vi "Query 1000.vi"(2 "error in (no error)":errorcluster, 3 "Parameters Query":T1) -> (0 "error out":errorcluster, 1 "Array":bool[](array[boolean]))   [LabVIEW 2015]
uses:
  C1G2_CommandControl.ctl
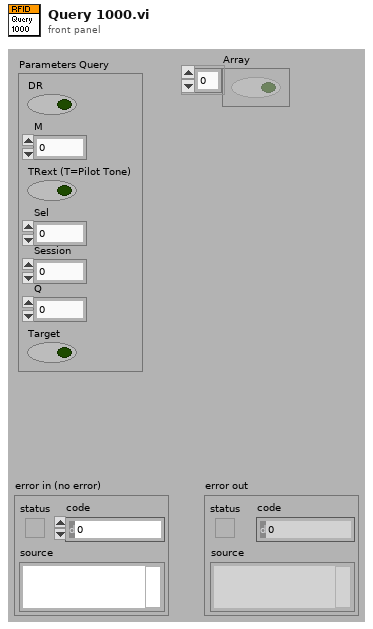
[diagram p1: front panel]
types:
  T1 = cluster{"DR":bool, "M":u16, "TRext (T=Pilot Tone)":bool, "Sel":u16, "Session":u16, "Q":u8, "Target":bool}
  T2 = typedef "C1G2_CommandControl.ctl" = u16
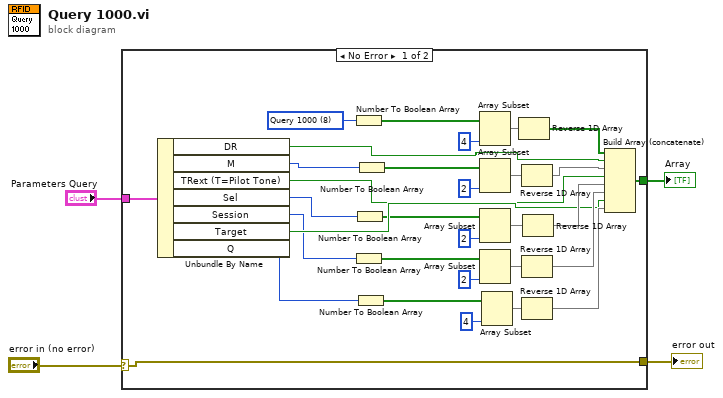
[diagram p0: block diagram]
diagram:
  n1 = case shown="No Error" "error in (no error)" {
    selector: "error in (no error)" -> [w5 w36]
    tunnel: [w35 _] -> w4
    tunnel: "Parameters Query" -> [w11 _]
    tunnel: [w5 w36] -> w1
    frame No Error {
      w6 = T2 8 items=["Select 1010"=10, "Query 1000"=8] ("Command")
      n2 = Unbundle By Name(w11) -> ("DR"=w14:bool, "M"=w7:u16, "TRext (T=Pilot Tone)"=w17:bool, "Sel"=w8:u16, "Session"=w9:u16, "Target"=w23:bool, "Q"=w10:u8)
      n3 = Number To Boolean Array(number=w6) -> (Boolean array=w13:bool[])
      n4 = Number To Boolean Array(number=w9) -> (Boolean array=w22:bool[])
      n5 = Number To Boolean Array(number=w8) -> (Boolean array=w19:bool[])
      n6 = Number To Boolean Array(number=w10) -> (Boolean array=w24:bool[])
      n7 = Number To Boolean Array(number=w7) -> (Boolean array=w16:bool[])
      n8 = Array Subset(array=w13, length=4) -> (w29:bool[])  [unwired: 1 in]
      n9 = Array Subset(array=w16, length=2) -> (w28:bool[])  [unwired: 1 in]
      n10 = Array Subset(array=w19, length=2) -> (w27:bool[])  [unwired: 1 in]
      n11 = Array Subset(array=w22, length=2) -> (w26:bool[])  [unwired: 1 in]
      n12 = Array Subset(array=w24, length=4) -> (w25:bool[])  [unwired: 1 in]
      n13 = Reverse 1D Array(array=w29) -> (reversed array=w30:bool[])
      n14 = Reverse 1D Array(array=w28) -> (reversed array=w31:bool[])
      n15 = Reverse 1D Array(array=w26) -> (reversed array=w33:bool[])
      n16 = Reverse 1D Array(array=w25) -> (reversed array=w34:bool[])
      n17 = Reverse 1D Array(array=w27) -> (reversed array=w32:bool[])
      n18 = Build Array (concatenate)(w30, w14, w31, w17, w32, w33, w23, w34) -> (w35:bool[])
    }
    frame Error {
    }
  }
  "Array" <- w4
  "error out" <- w1
